vi "Timestamp Interface.vi"(8 "Eventstring":string, 11 "Port index":i32) -> (1 "OutputRequest":T1)   [LabVIEW 2015]
doc: "Makes OutputRequest objects compatible with the DigitalOutput output driver, but specific to timestamp-only pulses.\n\n\"Port index\": Timestamp port number assigned during port reservation\n\"Eventstring\": String to send w/ timestamp"
uses:
  Typedefs/OutputRequest.ctl
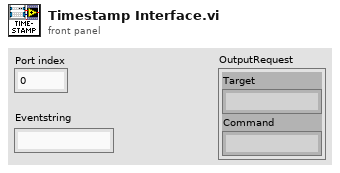
[diagram p1: front panel]
types:
  T1 = typedef "OutputRequest.ctl" = cluster{"Target":string, "Command":string}
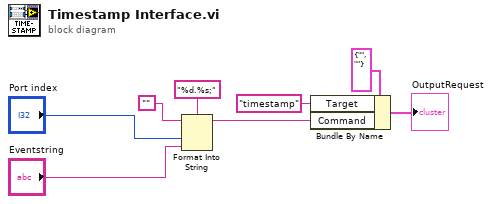
[diagram p0: block diagram]
diagram:
  n1 = Format Into String(format string="%d.%s;", initial string="", "Port index", "Eventstring") -> (resulting string=w5:string)  [unwired: 1 in, 1 out]
  n2 = Bundle By Name(cluster=T1 {"Target"="", "Command"=""} ("OutputRequest"), "Target"="timestamp", "Command"=w5) -> (→"OutputRequest":T1)
